vi "Puma_Ground_Control_Station_V2.1Smoothed.vi"(0 "?":refnum<visa-resource-name>="COM3", 1 "?":u32=9600, 9 "XON":u8=17 format="%.0x", 14 "XOFF":u8=19 format="%.0x", 15 "?":u32=10000, 21 "?":bool=TRUE, 24 "?":u8=10 format="%.0x", 25 "bsize":u32=4096) -> ()   [LabVIEW 2015]
doc: "The Advanced Serial Read and Write example performs a Serial Port Read, a Serial Port Write, or a combination of these actions while setting some advanced serial features like buffer size, termination characters, and XON/XOFF flow control. The user selects the actions (read or write) on the front panel. If both are selected, the VI will write the data first, read the data and then close the VISA session that is opened to the port. \n\nThe parameters set for the serial port must match the parameters of the connected instrument or device. In this example, the bytes to read parameter specifies the number of bytes that the serial port reads. If there were more bytes at the port than the number specified in bytes to read, those bytes would not be read. Also, if you specify to read more bytes than the number of bytes actually read, you might receive a timeout error message.\n\nINSTRUCTIONS:\n1) Select the serial resource and configuration parameters (baud rate, data bits, parity, stop bits, flow control).\n2) Termination character can be enabled and set. Also, set the required input buffer size prior to running the example.\n3) Select the operations to be performed. \n4) Connect the serial port to your device. If no device is available, perform a loopback test by doing one of the following. Short pins 2 and 3 on a RS-232 cable or short pin 4 to pin 8 and pin 5 to pin 9 on a RS-485/422 cable. \n5) Run the VI to see the data read. (The \"read string\" will match the \"string to write\" if a loopback test was performed.)\n\nThis example exposes several advanced features that you may need for your application. Not all applications need all the features shown in this example. The input buffer size is likely an important setting that you want to control in your application. This example expands upon the flow control option for XON and XOFF, allowing the user to choose those control characters. The timeout parameter has been brought to the front panel so a user can specify the time period the VISA Read will wait for the number of bytes to read before timing out. Also, the user has several controls for the termination character, which is discussed later.\n\nNote that you can press the write and read buttons and change the bytes to read parameters on the fly, while the example is running. However, you must stop the example to change the other configuration parameters after the example has started running, and then run again.\n\nSet the I/O buffer size slightly higher the amount of data you expect to receive. This is very important for applications that don't use flow control, as you may lose characters if the receive buffer overflows.\n\nSetting the timeout period ensures that the operation returns with a timeout error if the operation cannot be performed in the specified time period. \n\nSome devices require a termination character in order to identify the end of command strings. Some devices send a termination character to signify the end of data to be read. \n\nThis example shows how you can end the Read operation once a termination character is detected in the buffer and/or append a termination character at the end of the Write data. To enable the Read to end on a termination character, use the VISA Configure Serial Port or use the VISA Properties Serial End Mode for Reads, Termination Character Enable, and Termination Character. To end the Write with a termination character, use the VISA Properties Serial End Mode for Writes, the Send End Enable, and Termination Character. In this example, the same termination character is used for both the Read and the Write. You can specify two different characters for your application, if desired.\n\nYour application may require specific characters for the XON/XOFF Flow Control. You can specify these characters with the VISA Properties Flow Control XOFF Character and Flow Control XON Character. Note that if the standard XON and XOFF characters are used, then decimal 17 and 19 are unavailable for data values. Remember that using flow control and setting an adequate buffer size allow you to prevent buffer overflows."
uses:
  <vilib>/Instr/_visa.llb/VISA Configure Serial Port (Instr).vi
panel:
  in  "Fan Shutdown":bool
  in  "DValve / AV6-T":bool
  in  "Flight Control Board":bool
  in  "Safety":bool
  in  "Test Run":bool
  in  "Reset Control":bool
  in  "Primary Safety 2":bool
  out "?":bool
  out "Motors":cluster{dbl, dbl, dbl, dbl}(graph)={1000.0, 1000.0, 1000.0, 1000.0}
  in  "Pressure Transducers":T1(tab)
  out "?":cluster{dbl, dbl, dbl, dbl, dbl}(graph)
  out "?":cluster{dbl, dbl}(graph)
  in  "Thermocouples":T2(tab)
  out "?":cluster{dbl, dbl, dbl, dbl}(graph)
  out "?":cluster{dbl, dbl}(graph)
  out "fo-u":bool
  out "av5-m":bool
  out "fc-u":bool
  out "PT1-U > 5000 PSI":bool
  out "Takeoff Started":bool
  out "Iterations":i32
  out "Reset Triggered":bool
  in  "PixHawk":bool
  in  "XON 2":u8=17 format="%.0x"
  in  "XOFF 2":u8=19 format="%.0x"
  in  "?":bool=TRUE
  in  "bsize 2":u32=4096
  in  "?":u8=10 format="%.0x"
  in  "?":bool=TRUE
  in  "?":u32=10000
  in  "?":refnum<visa-resource-name>="COM3"
  in  "?":u32=9600
  out "Max Values":T3={20.764332288, 0.0, 0.0, 0.0, 0.0, 0.0, 0.0, 201.058, 25.138999999999953, 0.0, 57.16000000000008, 0.0, 8.920000000000016, 15.403999999999996}
  in  "Data Filename":string
  out "Offset 7":dbl=-251.3
  out "Multiplier 7":dbl=1.264
  out "Offset 6":dbl=-250.2
  out "Offset 5":dbl=-250.3
  out "Offset 4":dbl=-1253.0
  out "Offset 3":dbl=-250.9
  out "Offset 2":dbl=-249.8
  out "Offset 1":dbl=-251.0
  out "Multiplier 6":dbl=1.264
  out "Multiplier 5":dbl=1.277
  out "Multiplier 4":dbl=6.36
  out "Multiplier 3":dbl=1.274
  out "Multiplier 2":dbl=1.267
  out "Multiplier 1":dbl=1.277
  in  "Begin Checklist":bool
  out "Manual Abort Tested":bool
  out "Flight Control On":bool
  out "Reset Triggered 2":bool
  out "Primary Safety Active":bool
  out "Craft Triggered Softkill Active":bool
  out "Hardkill Active":bool
  out "ms":dbl=163640.0
  out "vcc 6":bool
  out "gnd 6":bool=TRUE
  out "TCp-2":bool
  out "vcc 5":bool
  out "gnd 5":bool=TRUE
  out "TCp-1":bool
  out "vcc 4":bool
  out "gnd 4":bool=TRUE
  out "TCpw-4":bool
  out "vcc 3":bool
  out "gnd 3":bool=TRUE
  out "TCpw-3":bool
  out "vcc 2":bool
  out "gnd 2":bool=TRUE
  out "TCpw-2":bool
  out "vcc":bool
  out "gnd":bool=TRUE
  out "TCpw-1":bool
  out "Engine 4":dbl=1000.0
  out "Engine 3":dbl=1000.0
  out "Engine 2":dbl=1000.0
  out "Engine 1":dbl=1000.0
  out "soft kill ind":bool
  out "dump fuel ind":bool
  out "abort ind":bool
  out "run ind":bool
  out "av6-t ind":bool
  out "Control input":bool
  out "return":bool
  out "Control (on/off)":bool
  out "PT5-M":dbl=-6.084000000000003
  out "PT2-M":dbl=-10.039999999999992
  out "PT2-U":dbl=-250.3
  out "PT1-U":dbl=-38.24000000000001
  out "PT3-M":dbl=-141.336
  out "PT1-M":dbl=9.934999999999945
  out "PT4-M":dbl=181.90299999999996
  out "TCp-2":dbl=-2.0
  out "TCp-1":dbl=-2.0
  out "TCpw-4":dbl=-2.0
  out "TCpw-3":dbl=-2.0
  out "TCpw-2":dbl=-2.0
  out "TCpw-1":dbl=-2.0
  out "Output":string="h:;"
  in  "?":enum32{"Test"}(tab)
  in  "Primary Safety":bool=TRUE
  in  "Soft Kill":bool
  in  "Simulate":bool
  in  "Reset FC":bool
  in  "Full Power":bool
  in  "Secondary Safety":bool=TRUE
  in  "Takeoff":bool
  in  "Calibrate":bool
  in  "Profile Selector":u16 max=9 step=1
  in  "abort":bool
  out "?":dbl(graph)=20.40794784
  in  "Send":bool=TRUE
  in  "Recieve":bool=TRUE
  in  "bytes to read 2":u32=1000
  out "?":u32=107
  out "?":string[](array[string])=["339", "205", "86", "191", "0", "190", "194", "-2.00", "-2.00", "-2.00", "-2.00", "-2.00", "-2.00", "555", "1000", "1000", "1000", "1000", "163640"]
  out "?":string[](array[string])=["p:339,205,86,191,0,190,194", "t:-2.00,-2.00,-2.00,-2.00,-2.00,-2.00", "v:555", "m:1000,1000,1000,1000", "h:", "s:163640", ""]
  out "Voltage Sensor":dbl=20.40794784
  in  "dump fuel":bool
  in  "?":enum32{"Ignore"}(tab)
  out "?":bool=TRUE
  out "String":string
  in  "String 3":string
  in  "?":bool=TRUE
  in  "tank iso":bool
  in  "Av-6Tt":bool
  in  "FC-U Toggle":bool
  in  "FOU":bool
  out "?":dbl(slide) scale=0.2..200.0
  out "FO-U":bool
  out "FC-U":bool
  out "AV6-T":bool
  out "AV1-T":bool
  out "AV3-T":bool
  out "AV4-T":bool
  out "AV5-T":bool
  out "AV2-T":bool
  # "Data From Craft:"
  # "FO-U"
  # "FC-U"
  # "receive"
  # "send"
  # "AV6-M"
  # "AV5-M"
  # "AV1-M"
  # "AV2-M"
  # "AV3-M"
  # "AV4-M"
  # "green=open - check thermocouple attachments\nred=short gnd - contact Power or GNC\nblue=short vcc - contact Power or GNC"
  # "Voltage"
  # "TCp2-M"
  # "Tcw1-E"
  # "TCp1-M"
  # "TCw4-E"
  # "TCw3-E"
  # "TCw2-E"
  # "PT4-M"
  # "PT1-M"
  # "PT3-M"
  # "PT1-U"
  # "PT2-U"
  # "PT2-M"
  # "PT5-M"
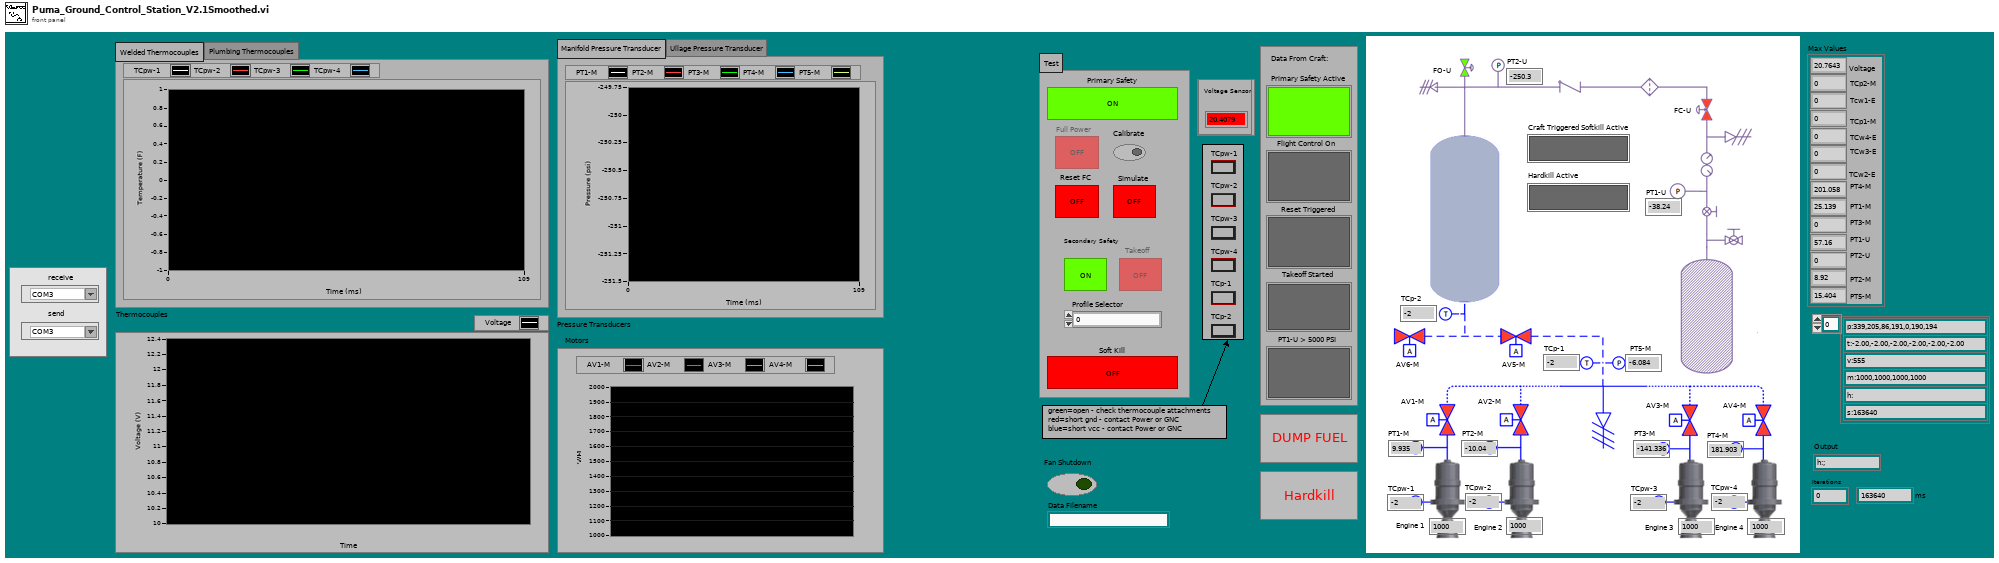
[diagram p1: front panel]
types:
  T1 = enum32{"Manifold Pressure Transducer", "Ullage Pressure Transducer"}
  T2 = enum32{"Welded Thermocouples", "Plumbing Thermocouples"}
  T3 = cluster{dbl, dbl, dbl, dbl, dbl, dbl, dbl, dbl, dbl, dbl, dbl, dbl, dbl, dbl}
  T4 = enum16{"open", "replace", "create", "open or create", "replace or create", "replace or create with confirmation"}
  T5 = cluster{"Output":dbl, dbl, dbl, dbl, dbl, dbl, dbl, "Output":dbl, "Output":dbl, "Output":dbl, "Output":dbl, "Output":dbl, "Output":dbl, "Output":dbl}
  T6 = cluster{"Output":dbl, "Output":dbl, "Output":dbl, "Output":dbl, "Output":dbl}
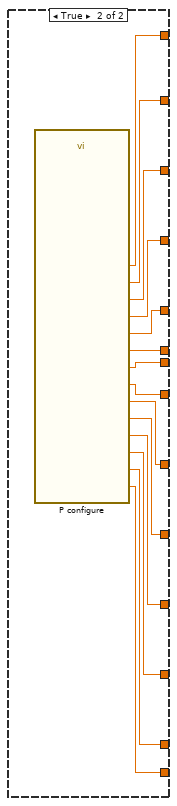
[diagram p3: hidden frame]
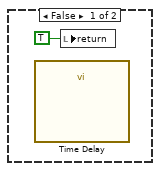
[diagram p13: hidden frame]
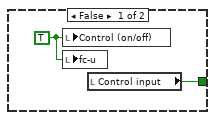
[diagram p17: hidden frame]
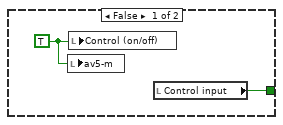
[diagram p19: hidden frame]
diagram:
  w2 = TRUE
  w1 = FALSE
  w51 = u16 16  # I/O Receive Buffer mask
  w75 = u16 16  # I/O Receive Buffer mask
  # "Comment"
  # "Set default values"
  n1 = while {
    stop <- FALSE stop-if-true
    n2 = case shown="False" "Calibrate" {
      tunnel: [w109 w123] -> w93
      tunnel: [w108 w122] -> w92
      tunnel: [w107 w121] -> w91
      tunnel: [w106 w120] -> w90
      tunnel: [w105 w119] -> w89
      tunnel: [w104 w118] -> w88
      tunnel: [w103 w117] -> w87
      tunnel: [w101 w116] -> w86
      tunnel: [w102 w115] -> w85
      tunnel: [w100 w114] -> w84
      tunnel: [w99 w113] -> w83
      tunnel: [w98 w112] -> w82
      tunnel: [w97 w111] -> w81
      tunnel: [w96 w110] -> w80
      frame False {
        n3 = local read "Multiplier 1"() -> (w109:dbl)
        n4 = local read "Multiplier 2"() -> (w108:dbl)
        n5 = local read "Multiplier 3"() -> (w107:dbl)
        n6 = local read "Multiplier 4"() -> (w106:dbl)
        n7 = local read "Multiplier 5"() -> (w105:dbl)
        n8 = local read "Multiplier 6"() -> (w104:dbl)
        n9 = local read "Multiplier 7"() -> (w103:dbl)
        n10 = local read "Offset 1"() -> (w101:dbl)
        n11 = local read "Offset 2"() -> (w102:dbl)
        n12 = local read "Offset 3"() -> (w100:dbl)
        n13 = local read "Offset 4"() -> (w99:dbl)
        n14 = local read "Offset 5"() -> (w98:dbl)
        n15 = local read "Offset 6"() -> (w97:dbl)
        n16 = local read "Offset 7"() -> (w96:dbl)
      }
      frame True {
        n17 = call "P configure.vi"() -> ("Multiplier 1"=w123:dbl, "Offset 1"=w116:dbl, "Multiplier 2"=w122:dbl, "Offset 2"=w115:dbl, "Multiplier 3"=w121:dbl, "Offset 6"=w111:dbl, "Offset 3"=w114:dbl, "Offset 7"=w110:dbl, "Multiplier 4"=w120:dbl, "Multiplier 7"=w117:dbl, "Multiplier 6"=w118:dbl, "Offset 5"=w112:dbl, "Multiplier 5"=w119:dbl, "Offset 4"=w113:dbl)  [unwired: 2 in]
      }
    }
    "Multiplier 1" <- w93
    "Multiplier 2" <- w92
    "Multiplier 3" <- w91
    "Multiplier 4" <- w90
    "Multiplier 5" <- w89
    "Offset 1" <- w86
    "Offset 2" <- w85
    "Offset 3" <- w84
    "Offset 4" <- w83
    "Offset 5" <- w82
    "Offset 6" <- w81
    "Multiplier 7" <- w87
    "Offset 7" <- w80
    "Multiplier 6" <- w88
  }
  n18 = while {
    stop <- FALSE stop-if-true
    n19 = local read "Control (on/off)"() -> (w126:bool)
    n20 = Wait Until Next ms Multiple(millisecond multiple=50) -> ()  [unwired: 1 out]
    n21 = case shown="True" w126 {
      frame False {
      }
      frame True {
        n22 = local read "dump fuel ind"() -> (w142:bool)
        n23 = local read "soft kill ind"() -> (w140:bool)
        n24 = local read "av6-t ind"() -> (w143:bool)
        n25 = local read "abort ind"() -> (w144:bool)
        n26 = local read "fc-u"() -> (w130:bool)
        n27 = local read "av5-m"() -> (w132:bool)
        n28 = local read "fo-u"() -> (w134:bool)
        n29 = local read "run ind"() -> (w141:bool)
        n30 = case shown="True" w140 {
          tunnel: [_ "Are you sure you want to Softkill?"] -> w135
          frame False {
          }
          frame True {
          }
        }
        n31 = case shown="True" w142 {
          tunnel: [_ "Are you sure you want to Dump Fuel?"] -> w137
          frame False {
          }
          frame True {
          }
        }
        n32 = case shown="True" w143 {
          tunnel: [_ "Are you sure you want to Open AV6-M?"] -> w138
          frame False {
          }
          frame True {
          }
        }
        n33 = case shown="True" w144 {
          tunnel: [_ "Are you sure you want to Abort?"] -> w139
          frame False {
          }
          frame True {
          }
        }
        n34 = case shown="True" w134 {
          tunnel: [_ "Are you sure you want to close FO-U?"] -> w133
          frame False {
          }
          frame True {
          }
        }
        n35 = case shown="True" w130 {
          tunnel: [_ "Are you sure you want to open FC-U?"] -> w129
          frame False {
          }
          frame True {
          }
        }
        n36 = case shown="True" w132 {
          tunnel: [_ "Are you sure you want to open AV5-M?"] -> w131
          frame False {
          }
          frame True {
          }
        }
        n37 = case shown="True" w141 {
          tunnel: [_ "Are you sure you want to Run?"] -> w136
          frame False {
          }
          frame True {
          }
        }
        n38 = Concatenate Strings(w135, w136, w137, w138, w139, w133, w131, w129) -> (w128:string)
        n39 = call "DialogBoxSubVI.vi"("Prompt"=w128) -> ("Boolean"=w127:bool)  [unwired: 9 in]
        n40 = case shown="True" w127 {
          frame False {
            n41 = call "Time Delay"() -> ()  [unwired: 11 in, 1 out]
            n42 = local write "return"(TRUE) -> ()
          }
          frame True {
            n43 = call "Time Delay2"() -> ()  [unwired: 11 in, 1 out]
            n44 = local write "return"(TRUE) -> ()
          }
        }
        n45 = local write "Control input"(w127) -> ()
      }
    }
  }
  n46 = call-poly "VISA Configure Serial Port"("VISA resource name"="?", "timeout (10sec)"="?", "termination char\n(0xA = '\\n' = LF)"="?", "Enable Termination\nChar (T)"="?", "baud rate (9600)"="?") -> ("VISA resource name out"=w64:refnum<visa-resource-name>, "error out"=w67:errorcluster)  [unwired: 5 in, 4 out]
  n47 = call-poly "VISA Configure Serial Port"("VISA resource name"="?", "timeout (10sec)"="?", "termination char\n(0xA = '\\n' = LF)"="?", "Enable Termination\nChar (T)"="?", "baud rate (9600)"="?") -> ("VISA resource name out"=w40:refnum<visa-resource-name>, "error out"=w43:errorcluster)  [unwired: 5 in, 4 out]
  n48 = case shown="True" "?" {
    selector: "?" -> [_ w157]
    tunnel: w64 -> [w155 w163]
    tunnel: w67 -> [w156 w162]
    tunnel: [w155 w161] -> w65
    tunnel: [w156 w160] -> w66
    tunnel: "?" -> [_ w158]
    frame False {
    }
    frame True {
      w159 = u16 2 items=["None", "LastBit", "TermChar", "Break"] ("Serial Settings:Serial End Mode for Writes")
      n49 = property class="Instr"(reference=w163, error in=w162, "Serial Settings:End Mode for Writes"=w159, "Message Based Settings:Send End Enable"=w157, "Message Based Settings:Termination Character"=w158) -> (reference out=w161:refnum<visa-resource-name>, error out=w160:errorcluster)
    }
  }
  n50 = case shown="True" "?" {
    selector: "?" -> [_ w166]
    tunnel: w40 -> [w164 w172]
    tunnel: w43 -> [w165 w171]
    tunnel: [w164 w170] -> w41
    tunnel: [w165 w169] -> w42
    tunnel: "?" -> [_ w167]
    frame False {
    }
    frame True {
      w168 = u16 2 items=["None", "LastBit", "TermChar", "Break"] ("Serial Settings:Serial End Mode for Writes")
      n51 = property class="Instr"(reference=w172, error in=w171, "Serial Settings:End Mode for Writes"=w168, "Message Based Settings:Send End Enable"=w166, "Message Based Settings:Termination Character"=w167) -> (reference out=w170:refnum<visa-resource-name>, error out=w169:errorcluster)
    }
  }
  n52 = property on="Secondary Safety" class="Bool (strict)"("Value"=w2) -> ()  [unwired: 2 in, 2 out]
  n53 = property on="Primary Safety" class="Bool (strict)"("Value"=w2) -> ()  [unwired: 2 in, 2 out]
  n54 = property on="Reset FC" class="Bool (strict)"("Value"=w1) -> ()  [unwired: 2 in, 2 out]
  n55 = property on="Simulate" class="Bool (strict)"("Value"=w1) -> ()  [unwired: 2 in, 2 out]
  n56 = property on="Craft Triggered Softkill Active" class="Bool (strict)"("Value"=w1) -> ()  [unwired: 2 in, 2 out]
  n57 = property on="Hardkill Active" class="Bool (strict)"("Value"=w1) -> ()  [unwired: 2 in, 2 out]
  n58 = property on="Takeoff Started" class="Bool (strict)"("Value"=w1) -> ()  [unwired: 2 in, 2 out]
  n59 = property on="FOU" class="Bool (strict)"("Value"=w1) -> ()  [unwired: 2 in, 2 out]
  n60 = property on="Soft Kill" class="Bool (strict)"("Value"=w1) -> ()  [unwired: 2 in, 2 out]
  n61 = property on="dump fuel" class="Bool (strict)"("Value"=w1) -> ()  [unwired: 2 in, 2 out]
  n62 = property on="abort" class="Bool (strict)"("Value"=w1) -> ()  [unwired: 2 in, 2 out]
  n63 = property on="Manual Abort Tested" class="Bool (strict)"("Value"=w1) -> ()  [unwired: 2 in, 2 out]
  n64 = Build Path(base path=path "C:/Users/Lunar Lion/Desktop/Puma_Test_Data" ("file path (use dialog)"), name or relative path="Data Filename") -> (appended path=w59:path)
  n65 = Build Array("PT4-M_a", "PT1-M_a", "PT3-M_a", "PT1-U_a", "PT2-U_a", "PT2-M_a", "PT5-M_a", "PT4-M", "PT1-M", "PT3-M", "PT1-U", "PT2-U", "PT2-M", "PT5-M", "TCp2-M", "TCw1-E", "TCp1-M", "TCw4-E", "TCw3-E", "TCw2-E", "Voltage", "Motor1", "Motor2", "Motor3", "Motor4", "Statestring") -> (w12:string[])
  n66 = VISA Set I/O Buffer Size(VISA resource name=w65, mask (16)=w75, size (4096)="bsize", error in (no error)=w66) -> (VISA resource name out=w71:refnum<visa-resource-name>, error out=w70:errorcluster)
  n67 = VISA Set I/O Buffer Size(VISA resource name=w41, mask (16)=w51, size (4096)="bsize 2", error in (no error)=w42) -> (VISA resource name out=w47:refnum<visa-resource-name>, error out=w46:errorcluster)
  n68 = Open/Create/Replace File(file path (use dialog)=w59, operation (0:open)=T4."replace or create with confirmation") -> (refnum out=w9:refnum<file>)  [unwired: 4 in, 2 out]
  n69 = Array To Spreadsheet String(array=w12, 3:"%s" ("format string")) -> (spreadsheet string=w10:string)  [unwired: 1 in]
  n70 = property class="Instr"(reference=w71, error in=w70, "Serial Settings:Flow Control XON Character"="XON", "Serial Settings:Flow Control XOFF Character"="XOFF") -> (reference out=w63:refnum<visa-resource-name>, error out=w62:errorcluster)
  n71 = property class="Instr"(reference=w47, error in=w46, "Serial Settings:Flow Control XON Character"="XON 2", "Serial Settings:Flow Control XOFF Character"="XOFF 2") -> (reference out=w39:refnum<visa-resource-name>)  [unwired: 1 out]
  n72 = Write to Text File(file (use dialog)=w9, text=w10) -> (refnum out=w8:refnum<file>)  [unwired: 2 in, 2 out]
  n73 = while {
    tunnel: w63 -> [w325]
    tunnel: w62 -> [w393]
    tunnel: [w304] -> w7
    tunnel: [w303] -> w61
    shift-right: [w493] -> _
    shift-left: _ -> [w492]
    shift-right: [w198] -> _
    shift-left: _ -> [w454]
    shift-right: [w462] -> _
    shift-left: _ -> [w463]
    shift-right: [w453] -> _
    shift-left: _ -> [w477]
    shift-right: [w219] -> _
    shift-left: _ -> [w475]
    shift-right: [w455] -> _
    shift-left: _ -> [w458]
    shift-right: ["Begin Checklist"] -> _
    shift-left: _ -> [w374]
    tunnel: w8 -> [w346]
    tunnel: [w343] -> w58
    shift-right: [w328] -> _
    shift-left: T3 {0.0, 0.0, 0.0, 0.0, 0.0, 0.0, 0.0, 0.0, 0.0, 0.0, 0.0, 0.0, 0.0, 0.0} -> [w327]
    tunnel: w39 -> [_]
    shift-right: [w215] -> _
    shift-left: _ -> [w218]
    shift-right: [w212] -> _
    shift-left: _ -> [w213]
    shift-right: [w209] -> _
    shift-left: _ -> [w210]
    i -> [w313]
    stop <- FALSE stop-if-true
    w240 = u32 13816530
    w244 = 120.0
    w250 = 1200.0
    w241 = u32 16776704
    w257 = 800.0
    # "The purpose of this indicator is not entirely clear"
    # "Hidden test run button."
    # "Hidden secondary safety."
    # "Hidden reset control button."
    # "Hidden flight control board button."
    # "Un-named indicator, hidden."
    # "Hidden dump valve indicator/button?"
    # "Hidden primary safety"
    # "Tabs for the main command buttons."
    # "Ignore tab with the two strings and indicator light."
    # "Above nominal thresholds:\n   All PTs except PT1-U: 800\n   TCpw-1 to 4: 1200\n   TCp-1 and 2: 120"
    # "The second String \nParsing Indicator"
    # "String Parsing Indicator control"
    # "ENSURE THE PTs ARE HOOKED UP PROPERLY"
    # "Here, if PT1-U indicates a pressure greater than 5000 psi,\nthe indicator represented in the case structure is turned green. Otherwise, it is turned red."
    # "FO-U Case"
    # "AV6 -T Case"
    # "AV5-T Case"
    # "AV5-T Toggle"
    n74 = case shown="True" FALSE {
      frame False {
      }
      frame True {
        w610 = FALSE
        n75 = local write "FOU"(TRUE) -> ()
        n76 = local write "AV1-T"(w610) -> ()
        n77 = local write "AV2-T"(w610) -> ()
        n78 = local write "AV3-T"(w610) -> ()
        n79 = local write "AV4-T"(w610) -> ()
        n80 = local write "FC-U Toggle"(w610) -> ()
        n81 = local write "tank iso"(w610) -> ()
      }
    }
    n82 = property on="abort" class="Bool (strict)"() -> ("Value"=w284:bool)  [unwired: 2 in, 2 out]
    n83 = local read "Voltage Sensor"() -> (w203:dbl)
    n84 = case shown="False" w284 {
      frame False {
        n85 = property on="Soft Kill" class="Bool (strict)"() -> ("Value"=w593:bool)  [unwired: 2 in, 2 out]
        n86 = case shown="True" w593 {
          frame False {
            n87 = property on="dump fuel" class="Bool (strict)"("DisabledEnum"=0) -> ()  [unwired: 2 in, 2 out]
          }
          frame True {
            n88 = property on="dump fuel" class="Bool (strict)"("DisabledEnum"=2) -> ()  [unwired: 2 in, 2 out]
          }
        }
      }
      frame True {
        n89 = property on="dump fuel" class="Bool (strict)"("DisabledEnum"=2) -> ()  [unwired: 2 in, 2 out]
      }
    }
    n90 = Greater?(x=w203, y=14.5) -> (0:w206:bool)
    n91 = Less Or Equal?(x=w203, y=16.8) -> (x <= y?=w299:bool)
    n92 = Less Or Equal?(x=w203, y=15.5) -> (x <= y?=w294:bool)
    n93 = Greater?(x=w203, y=15.5) -> (0:w298:bool)
    n94 = Greater?(x=w203, y=16.8) -> (0:w291:bool)
    n95 = Less Or Equal?(x=w203, y=17.0) -> (x <= y?=w292:bool)
    n96 = Greater?(x=w203, y=17.0) -> (0:w287:bool)
    n97 = And(x=w291, y=w292) -> (x .and. y?=w290:bool)
    n98 = And(x=w206, y=w294) -> (x .and. y?=w295:bool)
    n99 = And(x=w298, y=w299) -> (x .and. y?=w300:bool)
    n100 = Less Or Equal?(x=w203, y=14.5) -> (x <= y?=w204:bool)
    n101 = case shown="True" w295 {
      frame False {
      }
      frame True {
        n102 = property on="Voltage Sensor" class="DigNum (strict)"("NumText.TextColor"=u32 0) -> ()  [unwired: 2 in, 2 out]
        n103 = property on="Voltage Sensor" class="DigNum (strict)"("NumText.BGColor"=u32 16776704) -> ()  [unwired: 2 in, 2 out]
      }
    }
    n104 = case shown="True" w204 {
      frame False {
      }
      frame True {
        n105 = property on="Voltage Sensor" class="DigNum (strict)"("NumText.BG Color"=u32 16711680) -> ()  [unwired: 2 in, 2 out]
      }
    }
    n106 = case shown="True" w300 {
      frame False {
      }
      frame True {
        n107 = property on="Voltage Sensor" class="DigNum (strict)"("NumText.BGColor"=u32 6618880) -> ()  [unwired: 2 in, 2 out]
        n108 = property on="Voltage Sensor" class="DigNum (strict)"("NumText.TextColor"=u32 16777222) -> ()  [unwired: 2 in, 2 out]
      }
    }
    n109 = case shown="True" w290 {
      frame False {
      }
      frame True {
        n110 = property on="Voltage Sensor" class="DigNum (strict)"("NumText.BGColor"=u32 16776704) -> ()  [unwired: 2 in, 2 out]
        n111 = property on="Voltage Sensor" class="DigNum (strict)"("NumText.TextColor"=u32 16777222) -> ()  [unwired: 2 in, 2 out]
      }
    }
    n112 = case shown="True" w287 {
      frame False {
      }
      frame True {
        n113 = property on="Voltage Sensor" class="DigNum (strict)"("NumText.BGColor"=u32 16711704) -> ()  [unwired: 2 in, 2 out]
      }
    }
    n114 = Exclusive Or(1:w477, 2:"abort") -> (0:w479:bool)
    n115 = case shown="True" w479 {
      tunnel: [w674 w676] -> w453
      tunnel: w477 -> [w674 w675]
      frame False {
      }
      frame True {
        n116 = case shown="False" w675 {
          tunnel: [w677 FALSE ("T button?")] -> w676
          frame False {
            w678 = TRUE
            n117 = local write "abort ind"(w678) -> ()
            n118 = local write "Control (on/off)"(w678) -> ()
            n119 = local read "Control input"() -> (w677:bool)
          }
          frame True {
          }
        }
      }
    }
    n120 = Exclusive Or(1:w458, 2:"Soft Kill") -> (0:w456:bool)
    n121 = Exclusive Or(1:w475, 2:"dump fuel") -> (0:w476:bool)
    n122 = case shown="True" w456 {
      tunnel: [w664 w666] -> w455
      tunnel: w458 -> [w664 w665]
      frame False {
      }
      frame True {
        n123 = case shown="False" w665 {
          tunnel: [w667 _] -> w666
          frame False {
            w668 = TRUE
            n124 = local write "soft kill ind"(w668) -> ()
            n125 = local write "Control (on/off)"(w668) -> ()
            n126 = local read "Control input"() -> (w667:bool)
          }
          frame True {
          }
        }
      }
    }
    n127 = case shown="True" w476 {
      tunnel: [w669 w671] -> w219
      tunnel: w475 -> [w669 w670]
      frame False {
      }
      frame True {
        n128 = case shown="False" w670 {
          tunnel: [w673 _] -> w671
          frame False {
            w672 = TRUE
            n129 = local write "Control (on/off)"(w672) -> ()
            n130 = local write "dump fuel ind"(w672) -> ()
            n131 = local read "Control input"() -> (w673:bool)
          }
          frame True {
          }
        }
      }
    }
    n132 = Not(x="Secondary Safety") -> (.not. x?=w314:bool)
    n133 = property on="TCpw-1" class="DigNum (strict)"() -> ("Value"=w254:dbl)  [unwired: 2 in, 2 out]
    n134 = property on="TCpw-2" class="DigNum (strict)"() -> ("Value"=w249:dbl)  [unwired: 2 in, 2 out]
    n135 = property on="TCpw-3" class="DigNum (strict)"() -> ("Value"=w248:dbl)  [unwired: 2 in, 2 out]
    n136 = property on="TCpw-4" class="DigNum (strict)"() -> ("Value"=w247:dbl)  [unwired: 2 in, 2 out]
    n137 = property on="TCp-2" class="DigNum (strict)"() -> ("Value"=w242:dbl)  [unwired: 2 in, 2 out]
    n138 = property on="TCp-1" class="DigNum (strict)"() -> ("Value"=w243:dbl)  [unwired: 2 in, 2 out]
    n139 = property on="PT2-M" class="DigNum (strict)"() -> ("Value"=w267:dbl)  [unwired: 2 in, 2 out]
    n140 = property on="PT1-M" class="DigNum (strict)"() -> ("Value"=w268:dbl)  [unwired: 2 in, 2 out]
    n141 = property on="PT3-M" class="DigNum (strict)"() -> ("Value"=w266:dbl)  [unwired: 2 in, 2 out]
    n142 = property on="PT4-M" class="DigNum (strict)"() -> ("Value"=w265:dbl)  [unwired: 2 in, 2 out]
    n143 = property on="PT5-M" class="DigNum (strict)"() -> ("Value"=w259:dbl)  [unwired: 2 in, 2 out]
    n144 = property on="PT2-U" class="DigNum (strict)"() -> ("Value"=w258:dbl)  [unwired: 2 in, 2 out]
    n145 = And(x="Safety", y="Test Run") -> (x .and. y?=w508:bool)
    n146 = And(x=w314, y="Takeoff") -> (x .and. y?=w507:bool)
    n147 = Not(x="Secondary Safety") -> (.not. x?=w316:bool)
    n148 = Greater Or Equal?(x=w242, y=w244) -> (x >= y?=w245:bool)
    n149 = Greater Or Equal?(x=w243, y=w244) -> (x >= y?=w246:bool)
    n150 = Greater Or Equal?(x=w254, y=w250) -> (x >= y?=w255:bool)
    n151 = Greater Or Equal?(x=w249, y=w250) -> (x >= y?=w253:bool)
    n152 = Greater Or Equal?(x=w248, y=w250) -> (x >= y?=w252:bool)
    n153 = Greater Or Equal?(x=w247, y=w250) -> (x >= y?=w251:bool)
    n154 = Greater Or Equal?(x=w267, y=w257) -> (x >= y?=w263:bool)
    n155 = Greater Or Equal?(x=w268, y=w257) -> (x >= y?=w264:bool)
    n156 = Greater Or Equal?(x=w266, y=w257) -> (x >= y?=w262:bool)
    n157 = Greater Or Equal?(x=w265, y=w257) -> (x >= y?=w261:bool)
    n158 = Greater Or Equal?(x=w259, y=w257) -> (x >= y?=w260:bool)
    n159 = Greater Or Equal?(x=w258, y=w257) -> (x >= y?=w256:bool)
    n160 = case shown="True" "Recieve" {
      tunnel: w393 -> [w730 w735]
      tunnel: w325 -> [w731 w734]
      tunnel: [w730 w737] -> w303
      tunnel: [w731 w736] -> w304
      tunnel: [_ w733] -> _
      tunnel: [_ w732] -> w345
      frame False {
      }
      frame True {
        n161 = case "Read bytes from port." shown="No Error" w735 {
          selector: w735 -> [w740 w746]
          tunnel: [w743 w746] -> w737
          tunnel: [w744 w745] -> w736
          tunnel: w734 -> [w741 w745]
          tunnel: [w738 _] -> w733
          tunnel: [w738 _] -> w732
          frame No Error {
            n162 = VISA Read(VISA resource name=w741, byte count="bytes to read 2", error in (no error)=w740) -> (VISA resource name out=w744:refnum<visa-resource-name>, read buffer=w738:string, return count=→"?":u32, error out=w743:errorcluster)
          }
          frame Error {
          }
        }
      }
    }
    n163 = case shown="False" w316 {
      tunnel: [2 0] -> w315
      frame False {
      }
      frame True {
      }
    }
    n164 = Or(x=w507, y=w508) -> (x .or. y?=w482:bool)
    n165 = case shown="True" w245 {
      tunnel: w241 -> [_ w570]
      tunnel: w240 -> [w569 _]
      frame False {
        n166 = property on="TCp-2" class="DigNum (strict)"("NumText.BGColor"=w569) -> ()  [unwired: 2 in, 2 out]
      }
      frame True {
        n167 = property on="TCp-2" class="DigNum (strict)"("NumText.BGColor"=w570) -> ()  [unwired: 2 in, 2 out]
      }
    }
    n168 = case shown="True" w246 {
      tunnel: w241 -> [_ w572]
      tunnel: w240 -> [w571 _]
      frame False {
        n169 = property on="TCp-1" class="DigNum (strict)"("NumText.BGColor"=w571) -> ()  [unwired: 2 in, 2 out]
      }
      frame True {
        n170 = property on="TCp-1" class="DigNum (strict)"("NumText.BGColor"=w572) -> ()  [unwired: 2 in, 2 out]
      }
    }
    n171 = case shown="True" w255 {
      tunnel: w241 -> [_ w580]
      tunnel: w240 -> [w579 _]
      frame False {
        n172 = property on="TCpw-1" class="DigNum (strict)"("NumText.BGColor"=w579) -> ()  [unwired: 2 in, 2 out]
      }
      frame True {
        n173 = property on="TCpw-1" class="DigNum (strict)"("NumText.BGColor"=w580) -> ()  [unwired: 2 in, 2 out]
      }
    }
    n174 = case shown="True" w253 {
      tunnel: w241 -> [_ w578]
      tunnel: w240 -> [w577 _]
      frame False {
        n175 = property on="TCpw-2" class="DigNum (strict)"("NumText.BGColor"=w577) -> ()  [unwired: 2 in, 2 out]
      }
      frame True {
        n176 = property on="TCpw-2" class="DigNum (strict)"("NumText.BGColor"=w578) -> ()  [unwired: 2 in, 2 out]
      }
    }
    n177 = case shown="True" w252 {
      tunnel: w241 -> [_ w576]
      tunnel: w240 -> [w575 _]
      frame False {
        n178 = property on="TCpw-3" class="DigNum (strict)"("NumText.BGColor"=w575) -> ()  [unwired: 2 in, 2 out]
      }
      frame True {
        n179 = property on="TCpw-3" class="DigNum (strict)"("NumText.BGColor"=w576) -> ()  [unwired: 2 in, 2 out]
      }
    }
    n180 = case shown="True" w251 {
      tunnel: w241 -> [_ w574]
      tunnel: w240 -> [w573 _]
      frame False {
        n181 = property on="TCpw-4" class="DigNum (strict)"("NumText.BGColor"=w573) -> ()  [unwired: 2 in, 2 out]
      }
      frame True {
        n182 = property on="TCpw-4" class="DigNum (strict)"("NumText.BGColor"=w574) -> ()  [unwired: 2 in, 2 out]
      }
    }
    n183 = case shown="True" w263 {
      tunnel: w241 -> [_ w590]
      tunnel: w240 -> [w589 _]
      frame False {
        n184 = property on="PT2-M" class="DigNum (strict)"("NumText.BGColor"=w589) -> ()  [unwired: 2 in, 2 out]
      }
      frame True {
        n185 = property on="PT2-M" class="DigNum (strict)"("NumText.BGColor"=w590) -> ()  [unwired: 2 in, 2 out]
      }
    }
    n186 = case shown="True" w264 {
      tunnel: w241 -> [_ w592]
      tunnel: w240 -> [w591 _]
      frame False {
        n187 = property on="PT1-M" class="DigNum (strict)"("NumText.BGColor"=w591) -> ()  [unwired: 2 in, 2 out]
      }
      frame True {
        n188 = property on="PT1-M" class="DigNum (strict)"("NumText.BGColor"=w592) -> ()  [unwired: 2 in, 2 out]
      }
    }
    n189 = case shown="True" w262 {
      tunnel: w241 -> [_ w588]
      tunnel: w240 -> [w587 _]
      frame False {
        n190 = property on="PT3-M" class="DigNum (strict)"("NumText.BGColor"=w587) -> ()  [unwired: 2 in, 2 out]
      }
      frame True {
        n191 = property on="PT3-M" class="DigNum (strict)"("NumText.BGColor"=w588) -> ()  [unwired: 2 in, 2 out]
      }
    }
    n192 = case shown="True" w261 {
      tunnel: w241 -> [_ w586]
      tunnel: w240 -> [w585 _]
      frame False {
        n193 = property on="PT4-M" class="DigNum (strict)"("NumText.BGColor"=w585) -> ()  [unwired: 2 in, 2 out]
      }
      frame True {
        n194 = property on="PT4-M" class="DigNum (strict)"("NumText.BGColor"=w586) -> ()  [unwired: 2 in, 2 out]
      }
    }
    n195 = case shown="True" w260 {
      tunnel: w241 -> [_ w584]
      tunnel: w240 -> [w583 _]
      frame False {
        n196 = property on="PT5-M" class="DigNum (strict)"("NumText.BGColor"=w583) -> ()  [unwired: 2 in, 2 out]
      }
      frame True {
        n197 = property on="PT5-M" class="DigNum (strict)"("NumText.BGColor"=w584) -> ()  [unwired: 2 in, 2 out]
      }
    }
    n198 = case shown="True" w256 {
      tunnel: w241 -> [_ w582]
      tunnel: w240 -> [w581 _]
      frame False {
        n199 = property on="PT2-U" class="DigNum (strict)"("NumText.BGColor"=w581) -> ()  [unwired: 2 in, 2 out]
      }
      frame True {
        n200 = property on="PT2-U" class="DigNum (strict)"("NumText.BGColor"=w582) -> ()  [unwired: 2 in, 2 out]
      }
    }
    n201 = Exclusive Or(1:w454, 2:w482) -> (0:w481:bool)
    n202 = case shown="True" w481 {
      tunnel: [w680 w682] -> w198
      tunnel: w454 -> [w680 w681]
      frame False {
      }
      frame True {
        n203 = case shown="True" w681 {
          tunnel: [w684 _] -> w682
          frame False {
            w683 = TRUE
            n204 = local write "run ind"(w683) -> ()
            n205 = local write "Control (on/off)"(w683) -> ()
            n206 = local read "Control input"() -> (w684:bool)
          }
          frame True {
            w685 = FALSE
            n207 = local write "Test Run"(w685) -> ()
            n208 = local write "Control (on/off)"(w685) -> ()
            n209 = local write "Takeoff"(w685) -> ()
          }
        }
      }
    }
    "AV1-T" <- w198
    "AV4-T" <- w198
    "AV2-T" <- w198
    "AV3-T" <- w198
    n210 = case shown="True" "FC-U Toggle" {
      tunnel: [w551 w553] -> w209
      tunnel: w210 -> [w551 w552]
      frame False {
      }
      frame True {
        n211 = case shown="True" w552 {
          tunnel: [w554 _] -> w553
          frame False {
            w555 = TRUE
            n212 = local write "Control (on/off)"(w555) -> ()
            n213 = local write "fc-u"(w555) -> ()
            n214 = local read "Control input"() -> (w554:bool)
          }
          frame True {
            n215 = local write "FC-U Toggle"(FALSE) -> ()
          }
        }
      }
    }
    "FC-U" <- w209
    n216 = case shown="True" "tank iso" {
      tunnel: [w557 w559] -> w212
      tunnel: w213 -> [w557 w558]
      frame False {
      }
      frame True {
        n217 = case shown="True" w558 {
          tunnel: [w560 _] -> w559
          frame False {
            w561 = TRUE
            n218 = local write "av5-m"(w561) -> ()
            n219 = local write "Control (on/off)"(w561) -> ()
            n220 = local read "Control input"() -> (w560:bool)
          }
          frame True {
            n221 = local write "tank iso"(FALSE) -> ()
          }
        }
      }
    }
    "AV5-T" <- w212
    n222 = property on="Takeoff" class="Bool (strict)"("DisabledEnum"=w315) -> ()  [unwired: 2 in, 2 out]
    n223 = case shown="True" "FOU" {
      tunnel: [w563 w565] -> w215
      tunnel: w218 -> [w563 w564]
      frame False {
      }
      frame True {
        n224 = case shown="True" w564 {
          tunnel: [w566 _] -> w565
          frame False {
            w567 = TRUE
            n225 = local write "Control (on/off)"(w567) -> ()
            n226 = local read "Control input"() -> (w566:bool)
            n227 = local write "fo-u"(w567) -> ()
          }
          frame True {
            n228 = local write "FOU"(FALSE) -> ()
          }
        }
      }
    }
    "FO-U" <- w215
    n229 = Or(x=w453, y=w455) -> (x .or. y?=w480:bool)
    n230 = Or(x=w480, y=w219) -> (x .or. y?=w450:bool)
    n231 = Not(x=w450) -> (.not. x?=w286:bool)
    n232 = And(x=w286, y="Safety") -> (x .and. y?=w467:bool)
    n233 = And(x=w286, y="Test Run") -> (x .and. y?=w464:bool)
    n234 = And(x=w286, y="Secondary Safety") -> (x .and. y?=w466:bool)
    n235 = And(x=w286, y="Takeoff") -> (x .and. y?=w465:bool)
    n236 = local write "Safety"(w467) -> ()
    n237 = local write "Test Run"(w464) -> ()
    n238 = local write "Takeoff"(w465) -> ()
    n239 = Concatenate Strings(w345, "\n" ("string")) -> ()  [unwired: 1 out]
    n240 = Or(x=w467, y=w466) -> (x .or. y?=w470:bool)
    n241 = Or(x=w465, y=w464) -> (x .or. y?=w469:bool)
    n242 = Spreadsheet String To Array(delimiter (Tab)=";", format string="%d", spreadsheet string=w345, array type (2D Dbl)=string[] ["p:1234.1234.1234.1234,1234,1234", "t:1234,1234,1234"] ("Array of Strings 3")) -> (array=w545:string[])
    "?" <- w545
    n243 = Or(x=w470, y=w469) -> (x .or. y?=w468:bool)
    n244 = Or(x="Av-6Tt", y="DValve / AV6-T") -> (x .or. y?=w459:bool)
    n245 = Or(x="Reset Control", y="Reset FC") -> (x .or. y?=w494:bool)
    n246 = Or(x=w215, y=w198) -> (x .or. y?=w216:bool)
    n247 = local read "return"() -> (w473:bool)
    n248 = case shown="True" w459 {
      tunnel: [w658 w659] -> w462
      tunnel: w463 -> [w658 w660]
      frame False {
      }
      frame True {
        n249 = case shown="False" w660 {
          tunnel: [w662 _] -> w659
          frame False {
            w661 = TRUE
            n250 = local write "Control (on/off)"(w661) -> ()
            n251 = local write "av6-t ind"(w661) -> ()
            n252 = local read "Control input"() -> (w662:bool)
          }
          frame True {
            w663 = FALSE
            n253 = local write "Av-6Tt"(w663) -> ()
            n254 = local write "DValve / AV6-T"(w663) -> ()
          }
        }
      }
    }
    "AV6-T" <- w462
    "?" <- w462
    n255 = case shown="True" w198 {
      tunnel: [_ "o" ("write buffer")] -> w200
      tunnel: w492 -> [w698 w709]
      tunnel: [w699 w705] -> w493
      tunnel: w494 -> [w697 _]
      tunnel: [_ w702] -> w201
      frame False {
        n256 = case shown="False" w697 {
          tunnel: [w700 200.0] -> w699
          tunnel: w698 -> [w700 _]
          frame False {
          }
          frame True {
          }
        }
      }
      frame True {
        # "Send 'o' Takeoff"
        n257 = Subtract(x=w709, y=0.0) -> (x-y=w706:dbl)
        n258 = Greater Than 0?(x=w706) -> (x > 0?=w707:bool)
        n259 = case shown="False" w707 {
          selector: w707 -> [_ w714]
          tunnel: w706 -> [_ w715]
          tunnel: [w710 w715] -> w705
          frame False {
            n260 = local read "Takeoff Started"() -> (w711:bool)
            n261 = case shown="False" w711 {
              tunnel: [200.0 0.0] -> w710
              frame False {
              }
              frame True {
              }
            }
          }
          frame True {
            "Takeoff Started" <- w714
          }
        }
        n262 = property on="Profile Selector" class="DigNum (strict)"() -> ("Value"=w703:u16)  [unwired: 2 in, 2 out]
        n263 = Format Into String(w703) -> (resulting string=w702:string)  [unwired: 3 in, 1 out]
      }
    }
    "?" <- w493
    n264 = Or(x=w216, y=w468) -> (x .or. y?=w471:bool)
    n265 = Array Size(array=w545) -> (size(s)=w546:i32)
    n266 = for {
      N: w546 -> [_]
      tunnel: w545 -> [w755]
      tunnel: [w747] -> w491 mode=concatenating
      i -> [w754]
      n267 = Index Array(array=w755, index=w754) -> (element=w750:string)
      n268 = String Subset(string=w750, offset (0)=2) -> (substring=w748:string)  [unwired: 1 in]
      n269 = Spreadsheet String To Array(delimiter (Tab)=",", format string="%d", spreadsheet string=w748, array type (2D Dbl)=string[] ["p:1234.1234.1234.1234,1234,1234", "t:1234,1234,1234"] ("Array of Strings 3")) -> (array=w747:string[])
    }
    n270 = Or(x=w473, y=w471) -> (x .or. y?=w474:bool)
    n271 = And(x=w473, y=w474) -> (x .and. y?=w472:bool)
    n272 = case shown="True" w472 {
      tunnel: w198 -> [_ w621]
      tunnel: w455 -> [_ w624]
      tunnel: w454 -> [_ w623]
      tunnel: [_ w622] -> _
      tunnel: w219 -> [_ w622]
      tunnel: w453 -> [_ w620]
      tunnel: w215 -> [_ w618]
      tunnel: w212 -> [_ w617]
      tunnel: w209 -> [_ w614]
      frame False {
      }
      frame True {
        n273 = local read "fc-u"() -> (w615:bool)
        n274 = case shown="True" w621 {
          frame False {
            w656 = FALSE
            n275 = local write "return"(w656) -> ()
            n276 = local write "Control (on/off)"(w656) -> ()
            n277 = local write "Control input"(w656) -> ()
          }
          frame True {
            w657 = FALSE
            n278 = local write "return"(w657) -> ()
            n279 = local write "Control (on/off)"(w657) -> ()
            n280 = local write "Control input"(w657) -> ()
          }
        }
        n281 = case shown="True" w615 {
          tunnel: w614 -> [_ w631]
          frame False {
          }
          frame True {
            n282 = local write "fc-u"(FALSE) -> ()
            n283 = case shown="False" w631 {
              frame False {
                n284 = local write "FC-U Toggle"(FALSE) -> ()
              }
              frame True {
                n285 = local write "FC-U Toggle"(FALSE) -> ()
              }
            }
          }
        }
        n286 = local read "soft kill ind"() -> (w629:bool)
        n287 = local read "abort ind"() -> (w626:bool)
        n288 = local read "av6-t ind"() -> (w625:bool)
        n289 = local read "run ind"() -> (w627:bool)
        n290 = local read "dump fuel ind"() -> (w628:bool)
        n291 = local read "fo-u"() -> (w619:bool)
        n292 = case shown="True" w626 {
          tunnel: w620 -> [_ w648]
          frame False {
          }
          frame True {
            n293 = local write "abort"(w648) -> ()
            n294 = local write "abort ind"(FALSE) -> ()
          }
        }
        n295 = case shown="True" w629 {
          tunnel: w621 -> [_ _]
          tunnel: w624 -> [_ w650]
          frame False {
          }
          frame True {
            n296 = local write "Soft Kill"(w650) -> ()
            n297 = local write "soft kill ind"(FALSE) -> ()
          }
        }
        n298 = case shown="True" w627 {
          tunnel: w621 -> [_ w655]
          frame False {
          }
          frame True {
            n299 = local write "Takeoff"(w655) -> ()
            n300 = local write "Test Run"(w655) -> ()
            n301 = local write "run ind"(FALSE) -> ()
          }
        }
        n302 = case shown="True" w625 {
          tunnel: w623 -> [_ w643]
          frame False {
          }
          frame True {
            n303 = case shown="True" w643 {
              frame False {
                n304 = local write "Av-6Tt"(FALSE) -> ()
                n305 = local write "DValve / AV6-T"(FALSE) -> ()
              }
              frame True {
                n306 = local write "Av-6Tt"(FALSE) -> ()
                n307 = local write "DValve / AV6-T"(FALSE) -> ()
              }
            }
            n308 = local write "av6-t ind"(FALSE) -> ()
          }
        }
        n309 = case shown="True" w628 {
          tunnel: w622 -> [_ w652]
          frame False {
          }
          frame True {
            n310 = local write "dump fuel"(w652) -> ()
            n311 = local write "dump fuel ind"(FALSE) -> ()
          }
        }
        n312 = case shown="True" w619 {
          tunnel: w618 -> [_ w638]
          frame False {
          }
          frame True {
            n313 = case shown="True" w638 {
              frame False {
                n314 = local write "FOU"(FALSE) -> ()
              }
              frame True {
                n315 = local write "FOU"(FALSE) -> ()
              }
            }
            n316 = local write "fo-u"(FALSE) -> ()
          }
        }
        n317 = local read "av5-m"() -> (w616:bool)
        n318 = case shown="True" w616 {
          tunnel: w617 -> [_ w634]
          frame False {
          }
          frame True {
            n319 = case shown="False" w634 {
              frame False {
                n320 = local write "tank iso"(FALSE) -> ()
              }
              frame True {
                n321 = local write "tank iso"(FALSE) -> ()
              }
            }
            n322 = local write "av5-m"(FALSE) -> ()
          }
        }
      }
    }
    n323 = Not(x="Primary Safety") -> ()  [unwired: 1 out]
    n324 = case shown="False" "Primary Safety" {
      tunnel: [0 2] -> w312
      tunnel: [w604 FALSE] -> w309
      frame False {
        n325 = property on="Full Power" class="Bool (strict)"() -> ("Value"=w604:bool)  [unwired: 2 in, 2 out]
      }
      frame True {
      }
    }
    n326 = Not(x="Primary Safety") -> (.not. x?=w318:bool)
    n327 = case shown="False" "Simulate" {
      tunnel: w491 -> [w686 w687]
      tunnel: [w686 w687] -> w396
      tunnel: [_ w687] -> w490
      frame False {
      }
      frame True {
      }
    }
    "?" <- w396
    n328 = case shown="True" "PixHawk" {
      tunnel: [_ "y" ("write buffer")] -> w513
      frame False {
      }
      frame True {
        # "Send 'y' Turn on Pixhawk"
      }
    }
    n329 = case shown="True" w318 {
      tunnel: [_ "s" ("write buffer")] -> w517
      frame False {
      }
      frame True {
        # "Send 's' to disengage safety"
      }
    }
    n330 = case shown="True" w494 {
      tunnel: [_ "r" ("write buffer")] -> w515
      frame False {
      }
      frame True {
        # "Send 'r' Reset Flight Computer"
      }
    }
    n331 = case shown="True" "Simulate" {
      tunnel: [_ "p" ("write buffer")] -> w512
      frame False {
      }
      frame True {
        # "Send 'p' begin flight profile sim"
      }
    }
    n332 = Or(x="Flight Control Board", y="Full Power") -> (x .or. y?=w504:bool)
    n333 = case shown="True" w215 {
      tunnel: [_ "d"] -> w503
      frame False {
      }
      frame True {
      }
    }
    n334 = case shown="True" w504 {
      tunnel: [_ "z" ("write buffer")] -> w516
      frame False {
      }
      frame True {
        # "Send 'z' Turn on Power"
      }
    }
    n335 = case shown="True" w219 {
      tunnel: [_ "b" ("write buffer")] -> w499
      frame False {
      }
      frame True {
        # "Send 'b' Dump FUEL"
      }
    }
    n336 = case shown="True" w462 {
      tunnel: [_ "v" ("write buffer")] -> w500
      frame False {
      }
      frame True {
        # "Send 'v' Dump Valve"
      }
    }
    n337 = property on="Full Power" class="Bool (strict)"("Value"=w309) -> ()  [unwired: 2 in, 2 out]
    n338 = property on="Full Power" class="Bool (strict)"("DisabledEnum"=w312) -> ()  [unwired: 2 in, 2 out]
    n339 = case shown="True" w209 {
      tunnel: [_ "i"] -> w502
      frame False {
      }
      frame True {
      }
    }
    n340 = case shown="True" w212 {
      tunnel: [_ "t"] -> w501
      frame False {
      }
      frame True {
      }
    }
    n341 = case shown="True" w453 {
      tunnel: [_ "a" ("write buffer")] -> w498
      frame False {
      }
      frame True {
        # "Send 'a' ABORT"
        n342 = property on="Secondary Safety" class="Bool (strict)"("Value"=TRUE) -> ()  [unwired: 2 in, 2 out]
      }
    }
    n343 = case shown="True" w455 {
      tunnel: [_ "k" ("write buffer")] -> w514
      frame False {
      }
      frame True {
        # "Send 'k' softkill"
      }
    }
    n344 = case shown="True" "Fan Shutdown" {
      tunnel: [_ "f"] -> w199
      frame False {
      }
      frame True {
        # "Sends 'f' to shut off fan"
      }
    }
    n345 = Array Size(array=w396) -> (size(s)=w395:i32)
    n346 = Index Array(array=w490, index=0) -> (element=w489:string)
    "String" <- w489
    n347 = Index Array(array=w396, index=0) -> (element=w538:string)
    n348 = Index Array(array=w396, index=7) -> (element=w527:string)
    n349 = Index Array(array=w396, index=1) -> (element=w537:string)
    n350 = Index Array(array=w396, index=8) -> (element=w526:string)
    n351 = Index Array(array=w396, index=2) -> (element=w536:string)
    n352 = Index Array(array=w396, index=9) -> (element=w525:string)
    n353 = Index Array(array=w396, index=3) -> (element=w535:string)
    n354 = Index Array(array=w396, index=4) -> (element=w534:string)
    n355 = Index Array(array=w396, index=5) -> (element=w533:string)
    n356 = Index Array(array=w396, index=6) -> (element=w496:string)
    n357 = Index Array(array=w396, index=13) -> (element=w518:string)
    n358 = Index Array(array=w396, index=10) -> (element=w523:string)
    n359 = Index Array(array=w396, index=11) -> (element=w522:string)
    n360 = Index Array(array=w396, index=12) -> (element=w521:string)
    n361 = Index Array(array=w396, index=16) -> (element=w438:string)
    n362 = Index Array(array=w396, index=14) -> (element=w440:string)
    n363 = Index Array(array=w396, index=15) -> (element=w439:string)
    n364 = Index Array(array=w396, index=17) -> (element=w437:string)
    n365 = Fract/Exp String To Number(string=w538) -> (number=w335:dbl)  [unwired: 3 in, 1 out]
    n366 = Fract/Exp String To Number(string=w537) -> (number=w334:dbl)  [unwired: 3 in, 1 out]
    n367 = Fract/Exp String To Number(string=w536) -> (number=w333:dbl)  [unwired: 3 in, 1 out]
    n368 = Fract/Exp String To Number(string=w535) -> (number=w332:dbl)  [unwired: 3 in, 1 out]
    n369 = Fract/Exp String To Number(string=w518) -> (number=w280:dbl)  [unwired: 3 in, 1 out]
    n370 = Fract/Exp String To Number(string=w534) -> (number=w331:dbl)  [unwired: 3 in, 1 out]
    n371 = Fract/Exp String To Number(string=w533) -> (number=w330:dbl)  [unwired: 3 in, 1 out]
    n372 = Fract/Exp String To Number(string=w496) -> (number=w329:dbl)  [unwired: 3 in, 1 out]
    n373 = Fract/Exp String To Number(string=w438) -> (number=w225:dbl)  [unwired: 3 in, 1 out]
    n374 = Fract/Exp String To Number(string=w440) -> (number=w239:dbl)  [unwired: 3 in, 1 out]
    n375 = Fract/Exp String To Number(string=w439) -> (number=w234:dbl)  [unwired: 3 in, 1 out]
    n376 = Fract/Exp String To Number(string=w437) -> (number=w220:dbl)  [unwired: 3 in, 1 out]
    n377 = Decrement(x=w395) -> (x-1=w394:i32)
    n378 = Fract/Exp String To Number(string=w527) -> (number=w279:dbl)  [unwired: 3 in, 1 out]
    "TCpw-1" <- w279
    n379 = Fract/Exp String To Number(string=w526) -> (number=w278:dbl)  [unwired: 3 in, 1 out]
    "TCpw-2" <- w278
    n380 = Fract/Exp String To Number(string=w525) -> (number=w277:dbl)  [unwired: 3 in, 1 out]
    "TCpw-3" <- w277
    n381 = Fract/Exp String To Number(string=w523) -> (number=w276:dbl)  [unwired: 3 in, 1 out]
    "TCpw-4" <- w276
    n382 = Fract/Exp String To Number(string=w522) -> (number=w273:dbl)  [unwired: 3 in, 1 out]
    "TCp-1" <- w273
    n383 = Fract/Exp String To Number(string=w521) -> (number=w272:dbl)  [unwired: 3 in, 1 out]
    "TCp-2" <- w272
    n384 = local read "Multiplier 1"() -> (w361:dbl)
    n385 = local read "Multiplier 2"() -> (w359:dbl)
    n386 = local read "Multiplier 3"() -> (w357:dbl)
    n387 = local read "Multiplier 4"() -> (w355:dbl)
    n388 = local read "Multiplier 5"() -> (w353:dbl)
    n389 = local read "Multiplier 6"() -> (w350:dbl)
    n390 = Equal?(x=w489, y="String 3") -> (x = y?=→"?":bool)
    n391 = Index Array(array=w396, index=w394) -> (element=w399:string)
    n392 = Concatenate Strings("h" ("string"), ":" ("string"), w517, w516, w515, w503, w513, w512, w199, w514, w502, w501, w500, w498, w499, w201, w200, ";" ("string")) -> (w445:string)
    "Output" <- w445
    n393 = Divide(x=w239, y=10.0) -> (x/y=w237:dbl)
    n394 = Divide(x=w234, y=10.0) -> (x/y=w230:dbl)
    n395 = Divide(x=w225, y=10.0) -> (x/y=w227:dbl)
    n396 = Divide(x=w220, y=10.0) -> (x/y=w222:dbl)
    n397 = local read "Multiplier 7"() -> (w348:dbl)
    n398 = Subtract(x=w237, y=100.0) -> (x-y=→"Engine 1":dbl)
    n399 = Subtract(x=w227, y=100.0) -> (x-y=→"Engine 3":dbl)
    n400 = Subtract(x=w222, y=100.0) -> (x-y=→"Engine 4":dbl)
    n401 = Multiply(x=w335, y=w361) -> (x*y=w368:dbl)
    n402 = Multiply(x=w334, y=w359) -> (x*y=w367:dbl)
    n403 = Multiply(x=w333, y=w357) -> (x*y=w366:dbl)
    n404 = Multiply(x=w332, y=w355) -> (x*y=w365:dbl)
    n405 = Multiply(x=w331, y=w353) -> (x*y=w364:dbl)
    n406 = Multiply(x=w330, y=w350) -> (x*y=w363:dbl)
    n407 = Subtract(x=w230, y=100.0) -> (x-y=→"Engine 2":dbl)
    n408 = Bundle(w239, w234, w225, w220) -> (→"Motors":cluster{dbl, dbl, dbl, dbl})  [unwired: 1 in]
    n409 = Equal?(x=w279, y=-1.0) -> (x = y?=→"TCpw-1":bool)
    n410 = Equal?(x=w279, y=-3.0) -> (x = y?=→"vcc":bool)
    n411 = Equal?(x=w279, y=-2.0) -> (x = y?=→"gnd":bool)
    n412 = Equal?(x=w278, y=-2.0) -> (x = y?=→"gnd 2":bool)
    n413 = Equal?(x=w278, y=-3.0) -> (x = y?=→"vcc 2":bool)
    n414 = Equal?(x=w278, y=-1.0) -> (x = y?=→"TCpw-2":bool)
    n415 = Equal?(x=w277, y=-3.0) -> (x = y?=→"vcc 3":bool)
    n416 = Equal?(x=w277, y=-2.0) -> (x = y?=→"gnd 3":bool)
    n417 = Equal?(x=w277, y=-1.0) -> (x = y?=→"TCpw-3":bool)
    n418 = Equal?(x=w276, y=-2.0) -> (x = y?=→"gnd 4":bool)
    n419 = Equal?(x=w276, y=-1.0) -> (x = y?=→"TCpw-4":bool)
    n420 = Equal?(x=w276, y=-3.0) -> (x = y?=→"vcc 4":bool)
    n421 = Equal?(x=w273, y=-3.0) -> (x = y?=→"vcc 5":bool)
    n422 = Equal?(x=w273, y=-2.0) -> (x = y?=→"gnd 5":bool)
    n423 = Equal?(x=w273, y=-1.0) -> (x = y?=→"TCp-1":bool)
    n424 = Equal?(x=w272, y=-3.0) -> (x = y?=→"vcc 6":bool)
    n425 = Equal?(x=w272, y=-1.0) -> (x = y?=→"TCp-2":bool)
    n426 = Equal?(x=w272, y=-2.0) -> (x = y?=→"gnd 6":bool)
    n427 = Index Array(array=w396, index=18) -> (element=w339:string)
    n428 = Fract/Exp String To Number(string=w399) -> (number=→"ms":dbl)  [unwired: 3 in, 1 out]
    n429 = Equal?(x=w445, y=w339) -> (x = y?=w447:bool)
    n430 = Multiply(x=w329, y=w348) -> (x*y=w362:dbl)
    n431 = Search/Split String(string=w339, search string/char (-)="r") -> (offset of match=w385:i32)  [unwired: 1 in, 2 out]
    n432 = Search/Split String(string=w339, search string/char (-)="z") -> (offset of match=w387:i32)  [unwired: 1 in, 2 out]
    n433 = Search/Split String(string=w339, search string/char (-)="s") -> (offset of match=w389:i32)  [unwired: 1 in, 2 out]
    n434 = Search/Split String(string=w339, search string/char (-)="k") -> (offset of match=w451:i32)  [unwired: 1 in, 2 out]
    n435 = Search/Split String(string=w339, search string/char (-)="a") -> (offset of match=w392:i32)  [unwired: 1 in, 2 out]
    n436 = Search/Split String(string=w339, search string/char (-)="t") -> (offset of match=w381:i32)  [unwired: 1 in, 2 out]
    n437 = case shown="True" w447 {
      tunnel: [w613 _] -> w446
      tunnel: w445 -> [w613 _]
      frame False {
      }
      frame True {
      }
    }
    n438 = local read "Offset 1"() -> (w360:dbl)
    n439 = local read "Offset 2"() -> (w358:dbl)
    n440 = local read "Offset 3"() -> (w356:dbl)
    n441 = local read "Offset 4"() -> (w354:dbl)
    n442 = local read "Offset 5"() -> (w352:dbl)
    n443 = local read "Offset 6"() -> (w351:dbl)
    n444 = local read "Offset 7"() -> (w349:dbl)
    n445 = Greater Or Equal To 0?(x=w451) -> (x >= 0?=→"Craft Triggered Softkill Active":bool)
    n446 = Greater Or Equal To 0?(x=w392) -> (x >= 0?=w319:bool)
    "Hardkill Active" <- w319
    n447 = Greater Or Equal To 0?(x=w385) -> (x >= 0?=w324:bool)
    "Reset Triggered" <- w324
    n448 = Greater Or Equal To 0?(x=w387) -> (x >= 0?=w347:bool)
    "Flight Control On" <- w347
    n449 = Greater Or Equal To 0?(x=w381) -> (x >= 0?=w376:bool)
    n450 = Greater Or Equal To 0?(x=w389) -> (x >= 0?=w377:bool)
    "Primary Safety Active" <- w377
    n451 = Multiply(x=0.0069, y=w280) -> (x*y=w176:dbl)
    n452 = Bundle(w279, w278, w277, w276) -> (→"?":cluster{dbl, dbl, dbl, dbl})  [unwired: 1 in]
    n453 = Bundle(w273, w272) -> (→"?":cluster{dbl, dbl})  [unwired: 1 in]
    n454 = local read "Manual Abort Tested"() -> (w382:bool)
    n455 = local read "Reset Triggered 2"() -> (w383:bool)
    n456 = Add(x=w360, y=w368) -> (x+y=w197:dbl)
    n457 = Add(x=w358, y=w367) -> (x+y=w194:dbl)
    n458 = Add(x=w356, y=w366) -> (x+y=w191:dbl)
    n459 = Add(x=w354, y=w365) -> (x+y=w188:dbl)
    n460 = Add(x=w352, y=w364) -> (x+y=w185:dbl)
    n461 = Add(x=w351, y=w363) -> (x+y=w182:dbl)
    n462 = Add(x=w349, y=w362) -> (x+y=w179:dbl)
    n463 = Add(x=11.144, y=w176) -> (x+y=w175:dbl)
    n464 = call "N_Point_Running_Average.vi"("n"=5, "Input"=w191) -> ("Output"=w190:dbl)
    "PT3-M" <- w190
    n465 = call "N_Point_Running_Average.vi"("n"=5, "Input"=w182) -> ("Output"=w181:dbl)
    "PT2-M" <- w181
    n466 = call "N_Point_Running_Average.vi"("n"=5, "Input"=w179) -> ("Output"=w178:dbl)
    "PT5-M" <- w178
    n467 = call "N_Point_Running_Average.vi"("n"=5, "Input"=w188) -> ("Output"=w187:dbl)
    "PT1-U" <- w187
    n468 = call "N_Point_Running_Average.vi"("n"=5, "Input"=w185) -> ("Output"=w184:dbl)
    "PT2-U" <- w184
    n469 = call "N_Point_Running_Average.vi"("n"=5, "Input"=w175) -> ("Output"=w174:dbl)
    "Voltage Sensor" <- w174
    "?" <- w174
    n470 = call "N_Point_Running_Average.vi"("n"=5, "Input"=w194) -> ("Output"=w193:dbl)
    "PT1-M" <- w193
    n471 = call "N_Point_Running_Average.vi"("n"=5, "Input"=w197) -> ("Output"=w196:dbl)
    "PT4-M" <- w196
    n472 = Or(x=w382, y=w319) -> (x .or. y?=w379:bool)
    "Manual Abort Tested" <- w379
    n473 = Or(x=w383, y=w324) -> (x .or. y?=w378:bool)
    "Reset Triggered 2" <- w378
    n474 = local read "PT1-U"() -> (w306:dbl)
    n475 = Build Array(w335, w334, w333, w332, w331, w330, w329, w196, w193, w190, w187, w184, w181, w178, w279, w278, w277, w276, w273, w272, w174, w239, w234, w234, w220) -> (w342:dbl[])
    n476 = Bundle("Output"=w174, w279, w278, w277, w276, w273, w272, "Output"=w196, "Output"=w193, "Output"=w190, "Output"=w187, "Output"=w184, "Output"=w181, "Output"=w178) -> (w326:T5)  [unwired: 1 out]
    n477 = Subtract(x=w306, y=5000) -> (x-y=w307:dbl)
    n478 = Bundle("Output"=w187, "Output"=w184) -> (→"?":cluster{"Output":dbl, "Output":dbl})  [unwired: 1 in]
    n479 = Greater Than 0?(x=w307) -> (x > 0?=→"PT1-U > 5000 PSI":bool)
    n480 = Build Array(w379, w378, w347, w376, w377) -> (w375:bool[])
    n481 = Bundle("Output"=w193, "Output"=w181, "Output"=w190, "Output"=w196, "Output"=w178) -> (→"?":T6)  [unwired: 1 in]
    n482 = case shown="True" "Send" {
      tunnel: w393 -> [_ w722]
      tunnel: w446 -> [_ w721]
      tunnel: w325 -> [_ w720]
      frame False {
      }
      frame True {
        n483 = case shown="No Error" w722 {
          selector: w722 -> [w725 w729]
          tunnel: [w727 w728] -> _
          tunnel: [w726 w729] -> _
          tunnel: w721 -> [w724 _]
          tunnel: w720 -> [w723 w728]
          frame No Error {
            n484 = VISA Write(VISA resource name=w723, write buffer=w724, error in (no error)=w725) -> (VISA resource name out=w727:refnum<visa-resource-name>, error out=w726:errorcluster)  [unwired: 1 out]
          }
          frame Error {
          }
        }
      }
    }
    n485 = Array To Spreadsheet String(delimiter (Tab)="\t", array=w342, 3:"%d" ("format string")) -> (spreadsheet string=w323:string)
    n486 = Max & Min(x=w327, y=w326) -> (max(x,y)=w328:T3)  [unwired: 1 out]
    "Max Values" <- w328
    n487 = And Array Elements(Boolean array=w375) -> (logical AND=w371:bool)
    n488 = Search/Split String(string=w323, search string/char (-)="\r\n") -> (substring before match=w321:string)  [unwired: 1 in, 2 out]
    n489 = And(x=w374, y=w371) -> (x .and. y?=w373:bool)
    n490 = Concatenate Strings(w321, "\t" ("string"), w339, "\n" ("string")) -> (w337:string)
    n491 = Or(x=w374, y=w373) -> (x .or. y?=w372:bool)
    n492 = Write to Text File(file (use dialog)=w346, text=w337) -> (refnum out=w343:refnum<file>)  [unwired: 2 in, 2 out]
    n493 = Exclusive Or(1:w372, 2:"Begin Checklist") -> (0:w390:bool)
    n494 = case shown="True" w390 {
      frame False {
      }
      frame True {
        w612 = FALSE
        n495 = local write "Reset Triggered 2"(w612) -> ()
        n496 = local write "Manual Abort Tested"(w612) -> ()
      }
    }
    n497 = Wait Until Next ms Multiple(millisecond multiple=200) -> ()  [unwired: 1 out]
    "Iterations" <- w313
  }
  n498 = VISA Open(VISA resource name=refnum<visa-resource-name> "COM3") -> (VISA resource name=w5:refnum<visa-resource-name>, error out=w4:errorcluster)  [unwired: 4 in]
  n499 = VISA Close(VISA resource name=w5, error in (no error)=w4) -> ()  [unwired: 1 out]
  n500 = VISA Close(VISA resource name=w7, error in (no error)=w61) -> ()  [unwired: 1 out]
  n501 = Close File(refnum=w58) -> ()  [unwired: 1 in, 2 out]
